vi "Read Smooth Segments.vi"(8 "error in (no error)":errorcluster, 11 "Funnel Settings in":refnum<class "Funnel Settings.lvclass">) -> (0 "error out":errorcluster, 2 "Smooth Segments":dbl, 3 "Funnel Settings out":refnum<class "Funnel Settings.lvclass">)   [LabVIEW 2019, in "Funnel Settings.lvclass"]
uses:
  Funnel Settings.lvclass
  Funnel Settings.lvclass/Funnel Settings.ctl
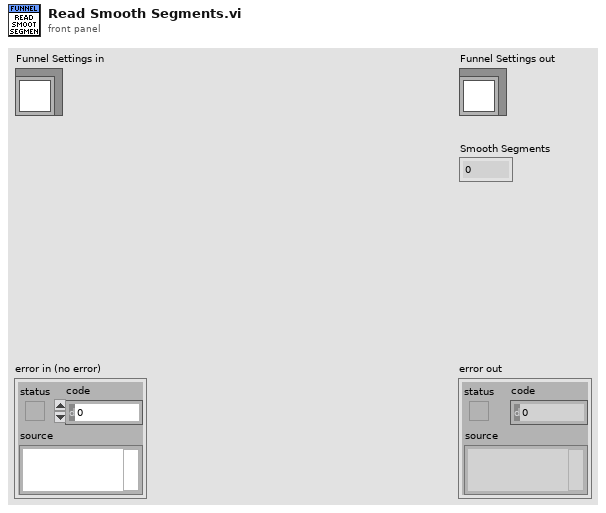
[diagram p1: front panel]
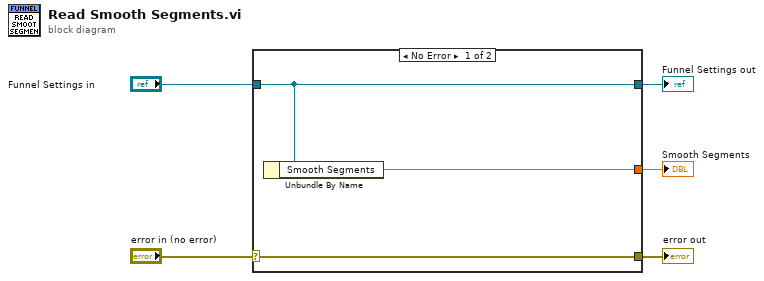
[diagram p0: block diagram]
diagram:
  n1 = case shown="No Error" "error in (no error)" {
    selector: "error in (no error)" -> [w8 w9]
    tunnel: [w8 w9] -> w4
    tunnel: [w7 w10] -> w2
    tunnel: "Funnel Settings in" -> [w7 w10]
    tunnel: [w6 _] -> w1
    frame No Error {
      n2 = Unbundle By Name(w7) -> ("Smooth Segments"=w6:dbl)
    }
    frame Error {
    }
  }
  "error out" <- w4
  "Funnel Settings out" <- w2
  "Smooth Segments" <- w1
